vi "daqio_Create_Event_Type.vi"(8 "error in (no error)":errorcluster, 9 "new Event Label":string, 10 "new Event Key":string, 11 "daq.io type in":T1={"daq.io ref"=refnum, "daq.io API Base"="http://dashboard.daq.io/api/v1", "Device Type Key"="", "Device Key"="", "Account ID"=""}) -> (0 "error out":errorcluster, 2 "actual Event Key written":string, 3 "daq.io type out":T1={"daq.io ref"=refnum, "daq.io API Base"="http://dashboard.daq.io/api/v1", "Device Type Key"="", "Device Key"="", "Account ID"=""})   [LabVIEW 2013, in "daqio minimal.lvlib"]
doc: "This VI uses defines a new Event on daq.io by creating a new event type. It does not perform automatic error checking. Using the \"Check and Autocreate\" function will perform a check before creating. Consider using this for automatic creation."
uses:
  _typedefs/daqio-Type.ctl
  <vilib>/httpClient/ClientHandle.ctl
  _typedefs/daqio-Event-Type-Min-Def.ctl
  daqio minimal.lvlib
  <vilib>/Easy HTTP Client/Easy HTTP.lvlib
  <vilib>/httpClient/LabVIEWHTTPClient.lvlib
panel:
  out "body":string
  out "JSON string":string
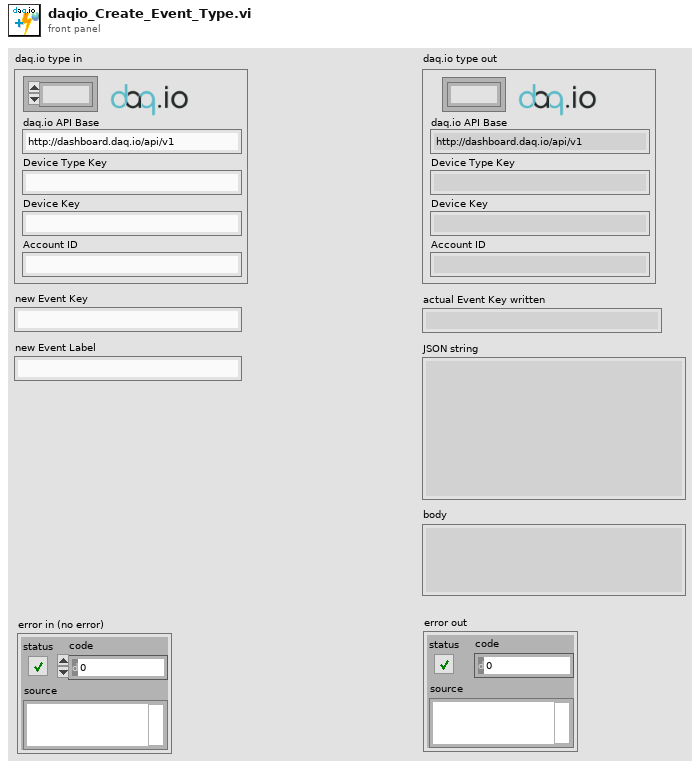
[diagram p1: front panel]
types:
  T1 = typedef "daqio minimal.lvlib/daqio-Type.ctl" = cluster{"daq.io ref":T2, "daq.io API Base":string, "Device Type Key":string, "Device Key":string, "Account ID":string}
  T2 = typedef "LabVIEWHTTPClient.lvlib/ClientHandle.ctl" = refnum<k1>
  T3 = typedef "daqio minimal.lvlib/daqio-Event-Type-Min-Def.ctl" = cluster{"device_type_id":string, "key":string, "label":string}
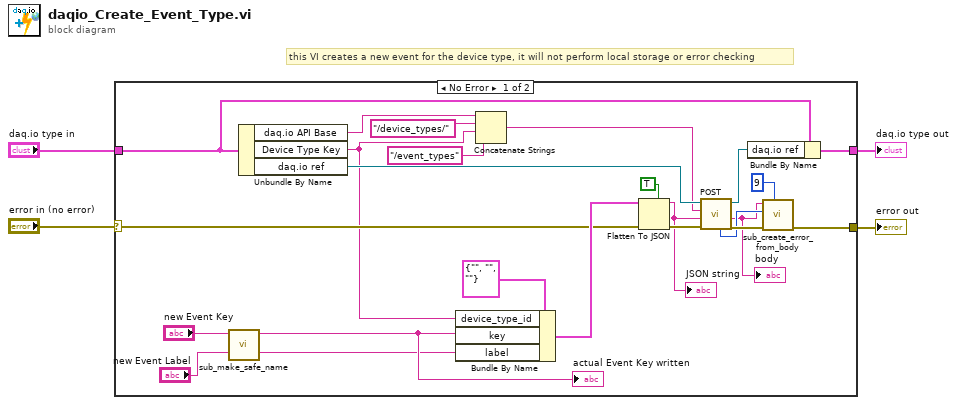
[diagram p0: block diagram]
diagram:
  # "this VI creates a new event for the device type, it will not perform local storage or error checking"
  n1 = case shown="No Error" "error in (no error)" {
    selector: "error in (no error)" -> [w22 w28]
    tunnel: [w19 w29] -> w4
    tunnel: [w8 w28] -> w3
    tunnel: "daq.io type in" -> [w18 w29]
    frame No Error {
      n2 = call "sub_make_safe_name.vi"("Input String"="new Event Key") -> ("Safe Output String"=w13:string)  [unwired: 10 in]
      "actual Event Key written" <- w13
      n3 = Unbundle By Name(w18) -> ("daq.io API Base"=w10:string, "Device Type Key"=w14:string, "daq.io ref"=w21:T2)
      n4 = Bundle By Name(cluster=T3 {"device_type_id"="", "key"="", "label"=""} ("Devices"), "device_type_id"=w14, "key"=w13, "label"="new Event Label") -> (w27:T3)
      n5 = Concatenate Strings(w10, "/device_types/" ("string"), w14, "/event_types" ("string")) -> (w16:string)
      n6 = Flatten To JSON(enable LabVIEW extensions? (T)=TRUE, anything=w27, error in (no error)=w22) -> (JSON string=w15:string, 11:w20:errorcluster)
      "JSON string" <- w15
      n7 = call <vilib>:"POST.vi"("error in (no error)"=w20, "data"=w15, "url"=w16, "client handle"=w21) -> ("error out"=w9:errorcluster, "body"=w6:string, "client handle out"=w17:T2, "HTTP Response Code"=w7:i32)  [unwired: 3 in, 1 out]
      "body" <- w6
      n8 = Bundle By Name(cluster=w18, "daq.io ref"=w17) -> (w19:T1)
      n9 = call "sub_create_error_from_body.vi"("error code"=9, "error in (no error)"=w9, "http code"=w7, "body"=w6) -> ("error out"=w8:errorcluster)  [unwired: 7 in]
    }
    frame Error {
    }
  }
  "error out" <- w3
  "daq.io type out" <- w4
